vi "GetBranches.vi"(6 "error in":errorcluster, 9 "Terminal in":refnum<class "Terminal.lvclass">) -> (0 "error out":errorcluster, 3 "Terminal out":refnum<class "Terminal.lvclass">, 4 "branches":i32, 5 "wire branched":bool)   [LabVIEW 2014, in "Terminal.lvclass"]
uses:
  Terminal.lvclass
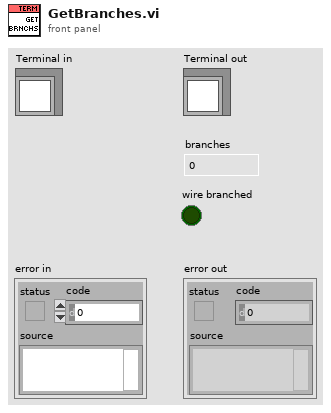
[diagram p1: front panel]
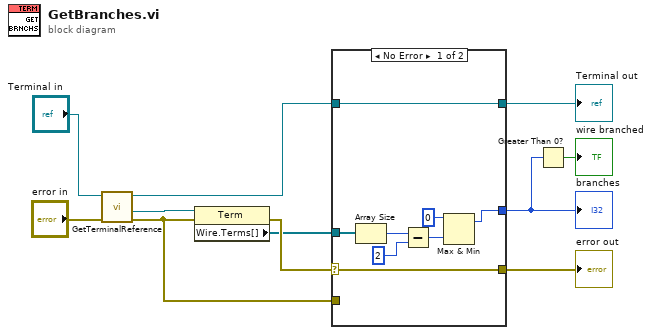
[diagram p0: block diagram]
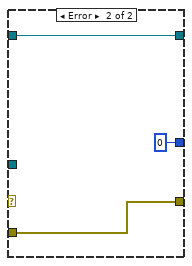
[diagram p2: hidden frame]
diagram:
  n1 = call "GetTerminalReference.vi"("error in"="error in", "Terminal in"="Terminal in") -> ("error out"=w8:errorcluster, "reference"=w9:refnum<vi>, "Terminal out"=w6:refnum<class "Terminal.lvclass">)  [unwired: 7 in]
  n2 = property class="Term"(reference=w9, error in=w8) -> (error out=w4:errorcluster, "Wire.Terms[]"=w3:refnum<vi>[])  [unwired: 1 out]
  n3 = case shown="No Error" w4 {
    selector: w4 -> [w18 _]
    tunnel: w8 -> [_ w21]
    tunnel: [w19 w22] -> w7
    tunnel: w6 -> [w19 w22]
    tunnel: [w18 w21] -> w5
    tunnel: [w13 0 ("index of element")] -> w1
    tunnel: w3 -> [w17 _]
    frame No Error {
      n4 = Array Size(array=w17) -> (size(s)=w16:i32)
      n5 = Subtract(x=w16, y=2) -> (x-y=w14:i32)
      n6 = Max & Min(x=0, y=w14) -> (max(x,y)=w13:i32)  [unwired: 1 out]
    }
    frame Error {
    }
  }
  "error out" <- w5
  "Terminal out" <- w7
  "branches" <- w1
  n7 = Greater Than 0?(x=w1) -> (x > 0?=→"wire branched":bool)
